vi "Get Ordered List of Files.vi"(5 "Left/Right":T1(ring), 6 "pattern":string, 7 "Split string":string, 8 "Error In":errorcluster, 11 "Folder Path":path) -> (0 "Error Out":errorcluster, 1 "Root String":string, 3 "Folder Path dup":path, 4 "Ordered File Paths":path[](array[path]))   [LabVIEW 2021, in "Files.lvlib"]
uses:
  Files.lvlib
  <userlib>/_OpenG.lib/array/array.llb/Reorder 1D Array2 (String)__ogtk.vi
  Strings/Strings.lvlib
  <userlib>/_OpenG.lib/file/file.llb/openg_file.lvlib
  <userlib>/_OpenG.lib/array/array.llb/openg_array.lvlib
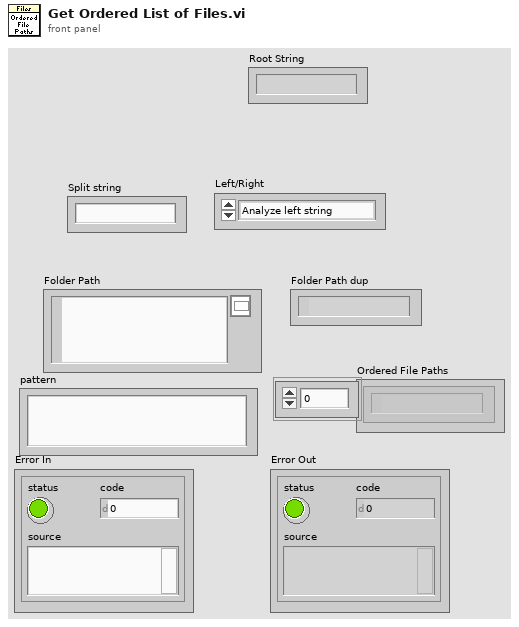
[diagram p1: front panel]
types:
  T1 = enum16{"Analyze left string", "Analyze right string"}
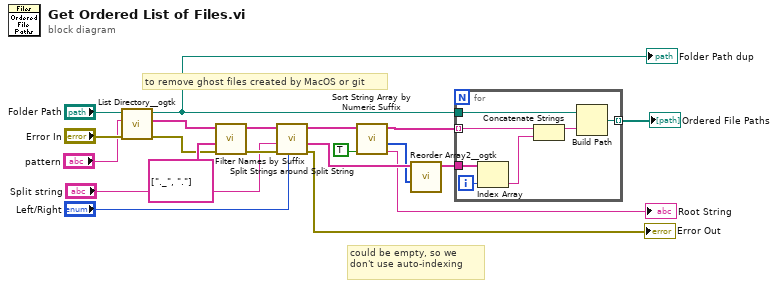
[diagram p0: block diagram]
diagram:
  # "could be empty, so we don't use auto-indexing"
  # "to remove ghost files created by MacOS or git"
  n1 = call <userlib>:"List Directory__ogtk.vi"("error in (no error)"="Error In", "pattern"="pattern", "directory path"="Folder Path") -> ("error out"=w11:errorcluster, "file names"=w17:string[], "dup directory path"=w18:path)  [unwired: 1 in, 1 out]
  "Folder Path dup" <- w18
  n2 = call "Filter Names by Suffix.vi"("Error In"=w11, "Ignore File Suffix Array"=string[] ["._", "."], "File Names"=w17) -> ("Error Out"=w8:errorcluster, "Filtered File Names"=w10:string[])  [unwired: 7 in]
  n3 = call "Split Strings around Split String.vi"("Left/Right"="Left/Right", "error in (no error)"=w8, "Split string"="Split string", "Filtered File Names in"=w10) -> ("error out"=→"Error Out":errorcluster, "Residual Strings"=w4:string[], "Filtered File Names out"=w9:string[])  [unwired: 5 in]
  n4 = call "Sort String Array by Numeric Suffix.vi"("Ignore File Extension"=TRUE, "String Array"=w9) -> ("Root String"=→"Root String":string, "Sorted Indices"=w3:i32[], "Sorted String Array"=w16:string[])  [unwired: 7 in]
  n5 = call-poly <userlib>:"Reorder Array2__ogtk.vi"("indices"=w3, "array"=w4) -> ("reordered array"=w2:string[])  [unwired: 9 in]
  n6 = for {
    tunnel: w16 -> [w27] mode=indexing
    tunnel: w18 -> [w26]
    tunnel: [w25] -> w19 mode=indexing
    tunnel: w2 -> [w24]
    i -> [w23]
    n7 = Index Array(array=w24, index=w23) -> (element=w21:string)
    n8 = Concatenate Strings(w27, w21) -> (w22:string)
    n9 = Build Path(base path=w26, name or relative path=w22) -> (appended path=w25:path)
  }
  "Ordered File Paths" <- w19
